vi "Get Qualified Name.vi"(8 "error in (no error)":errorcluster, 10 "separator (dot)":string caption="separator", 11 "SMO":refnum<class "SMO.lvclass">) -> (0 "error out":errorcluster, 1 "Reserved Qualified Name":string, 2 "Qualified Name":string, 3 "SMO out":refnum<class "SMO.lvclass">)   [LabVIEW 2021, in "smo.lvlib" / "SMO.lvclass"]
uses:
  SMO.lvclass
  SMO.lvclass/SMO.ctl
  Support/Attribute.Owner/Attribute.Owner.lvclass/Attribute.Owner.ctl
  Support/Attribute.Identity/Attribute.Identity.lvclass/Attribute.Identity.ctl
  Private/GetVariant(Attr).vi
  Support/Attribute.Owner/Read Lineage.vi
  Support/Attribute.Identity/Read UniqueName.vi
  Support/Attribute.Identity/Read Given Name.vi
  Support/Attribute.Identity/Read ProspectiveOwner.vi
  Private/ReftoDVR--SMO.vi
  Support/Attribute.Owner/Attribute.Owner.lvclass
  Support/Attribute.Identity/Attribute.Identity.lvclass
panel:
  # "This method is deprecated (as a Public API) but kept public for\nbackward-compatibility.\nUse the \"GetQualifiedName.vi\" method instead of \"Get Qualified Name.vi\""
  # "For instructions on how to use the JKI State Machine Objects, examples and video tutorials, visit:\nhttp://jki.net/state-machine-objects/\n\nJKI State Machine Objects™\nhttp://jki.net/state-machine-objects/\nCopyright (C) 2005-2015, JKI <info@jki.net>\nALL RIGHTS RESERVED"
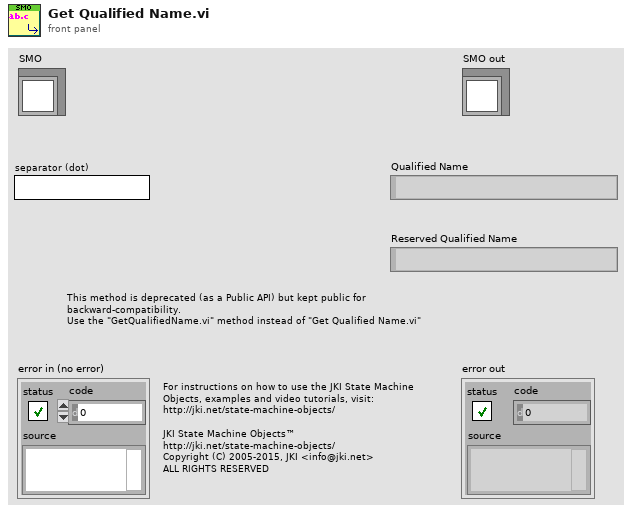
[diagram p1: front panel]
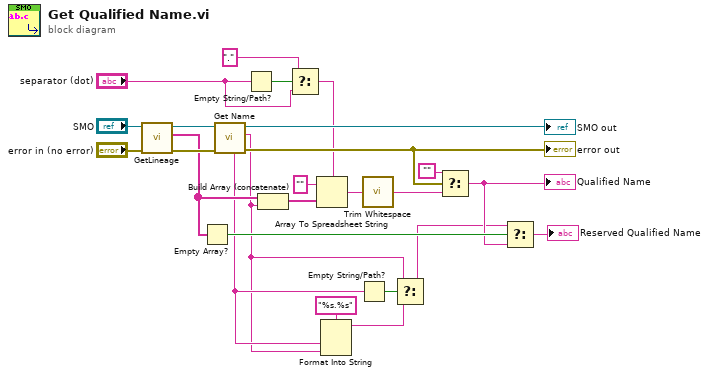
[diagram p0: block diagram]
diagram:
  n1 = call "GetLineage.vi"("error in (no error)"="error in (no error)", "SMO in"="SMO") -> ("error out"=w13:errorcluster, "Lineage"=w7:string[], "SMO out"=w11:refnum<class "SMO.lvclass">)  [unwired: 7 in]
  n2 = Empty Array?(array=w7) -> (empty?=w6:bool)
  n3 = call "Get Name.vi"("error in (no error)"=w13, "SMO"=w11) -> ("error out"=w23:errorcluster, "Name"=w1:string, "SMO out"=→"SMO out":refnum<class "SMO.lvclass">, "Prospective Owner"=w2:string)  [unwired: 5 in, 1 out]
  "error out" <- w23
  n4 = Empty String/Path?(string/path="separator (dot)") -> (empty?=w18:bool)
  n5 = Build Array (concatenate)(w7, w1) -> (w22:string[])
  n6 = Select(t="." ("delimiter (Tab)"), s=w18, f="separator (dot)") -> (s? t:f=w15:string)
  n7 = Array To Spreadsheet String(delimiter (Tab)=w15, array=w22, 3:"" ("format string")) -> (spreadsheet string=w20:string)
  n8 = Format Into String(format string="%s.%s", w2, w1) -> (resulting string=w9:string)  [unwired: 2 in, 1 out]
  n9 = Empty String/Path?(string/path=w2) -> (empty?=w10:bool)
  n10 = call <vilib>:"Trim Whitespace.vi"("string"=w20) -> ("trimmed string"=w19:string)  [unwired: 1 in]
  n11 = Select(t=w1, s=w10, f=w9) -> (s? t:f=w4:string)
  n12 = Select(t="", s=w23, f=w19) -> (s? t:f=w5:string)
  "Qualified Name" <- w5
  n13 = Select(t=w4, s=w6, f=w5) -> (s? t:f=→"Reserved Qualified Name":string)
